vi "sub vi - AI USB4704 (3)  Close Task v1.vi"(0 "TASK USB 0":i32, 5 "TASK USB 1":i32, 7 "TASK USB 2":i32) -> ()   [LabVIEW 2013]
panel:
  out "error array":errorcluster[](array[cluster])
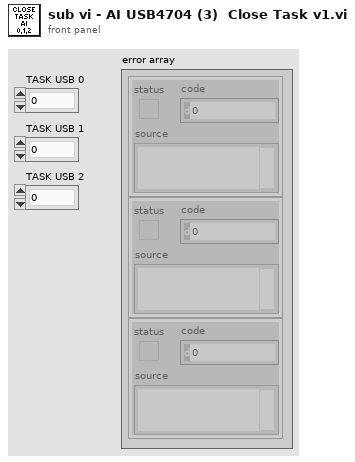
[diagram p1: front panel]
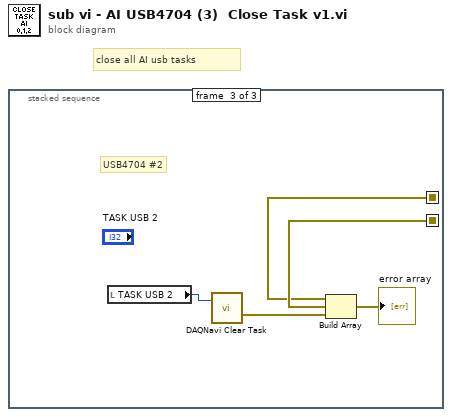
[diagram p0: block diagram]
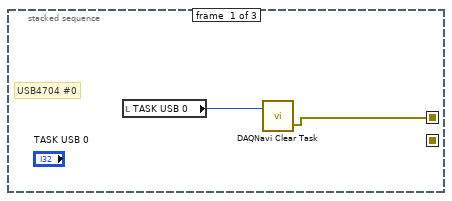
[diagram p2: hidden frame]
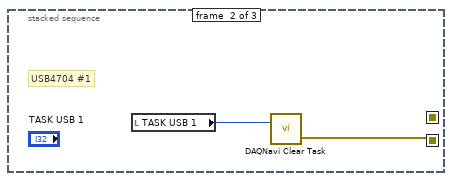
[diagram p3: hidden frame]
diagram:
  # "close all AI usb tasks"
  n1 = stacked-sequence {
    seq-local: [w1 _ _] -> [_ _ w6]
    seq-local: [_ w3 _] -> [_ _ w7]
    frame #0 {
      # "USB4704 #0"
      n2 = local read "TASK USB 0"() -> (w2:i32)
      n3 = call <userlib>:"DAQNavi Clear Task.vi"("task in"=w2) -> ("error out"=w1:errorcluster)  [unwired: 1 in, 1 out]
    }
    frame #1 {
      # "USB4704 #1"
      n4 = local read "TASK USB 1"() -> (w4:i32)
      n5 = call <userlib>:"DAQNavi Clear Task.vi"("task in"=w4) -> ("error out"=w3:errorcluster)  [unwired: 1 in, 1 out]
    }
    frame #2 {
      # "USB4704 #2"
      n6 = local read "TASK USB 2"() -> (w9:i32)
      n7 = call <userlib>:"DAQNavi Clear Task.vi"("task in"=w9) -> ("error out"=w8:errorcluster)  [unwired: 1 in, 1 out]
      n8 = Build Array(w6, w7, w8) -> (→"error array":errorcluster[])
    }
  }
